vi "Test Customer Pick Up Order Broadcasts Order Item.vi"(8 "error in (no error)":errorcluster, 11 "Customer Test in":refnum<class "Customer Test.lvclass">) -> (0 "error out":errorcluster, 3 "Customer Test out":refnum<class "Customer Test.lvclass">)   [LabVIEW 2020, in "Customer Test.lvclass"]
uses:
  Customer Test.lvclass
  C:/Program Files (x86)/National Instruments/LabVIEW 2020/vi.lib/Asteme/LUnit/Test Case.lvclass
  Customer/Customer.lvclass
  C:/Program Files (x86)/National Instruments/LabVIEW 2020/vi.lib/Asteme/Triarc Framework/Process/Process.lvclass
  Support/Beverages/Beverage/Beverage.lvclass
  <vilib>/Asteme/Triarc Framework/Process/Process.lvclass/Process.ctl
  <vilib>/Asteme/LUnit/Test Case.lvclass/Test Case.ctl
  <vilib>/Asteme/LUnit/LUnit Assertion Result.lvclass/LUnit Assertion Result.ctl
  <vilib>/Asteme/Triarc Framework Test Suite/Support/Execution timer.vi
  <vilib>/Asteme/Triarc Framework/Process/Private/SubVIs/Wait for finish.vi
  <vilib>/Asteme/Triarc Framework/Process/Protected/Messaging/Enqueue Message.vi
  <vilib>/Asteme/Triarc Framework/Process/Private/SubVIs/Set Lifecycle State.vi
  <vilib>/Asteme/Triarc Framework/Process/Public/Lifecycle/Get Lifecycle State.vi
  <vilib>/Asteme/LUnit/Palette/Pass.vi
  <vilib>/Asteme/LUnit/Palette/Fail.vi
  <vilib>/Asteme/LUnit/Variant to string.vi
  <vilib>/Asteme/LUnit/Set Assertion Type.vi
  <vilib>/Utility/error.llb/Clear Errors.vi
  <vilib>/Asteme/LUnit/Add test result.vi
  <vilib>/Asteme/LUnit/LUnit Write Passed.vi
  <vilib>/Asteme/LUnit/LUnit Get Test Case.vi
  <vilib>/Asteme/LUnit/Assertion Result/LUnit Get Test Name.vi
  <vilib>/Asteme/LUnit/LUnit Write Message.vi
  <vilib>/Asteme/LUnit/LUnit Write Description.vi
  <vilib>/Asteme/LUnit/LUnit Write Assertion Type.vi
  <vilib>/Asteme/LUnit/Read Test Case Name.vi
  <vilib>/Asteme/Triarc Framework Test Suite/Support/Event Helpers/Dequeue Event Message.vi
  <vilib>/Utility/error.llb/Error Cluster From Error Code.vi
  <vilib>/Utility/Data Type/Get Type Information.vi
  <vilib>/Utility/LVClass/Get LV Class Name.vi
  <vilib>/Asteme/LUnit/LUnit Assertion Result.lvclass
  <vilib>/Asteme/Triarc Framework/Process/Process.lvclass
  <vilib>/Asteme/Triarc Framework Test Suite/Support/Event Helpers/Event Helpers.lvlib
  <vilib>/Asteme/LUnit/Test Case.lvclass
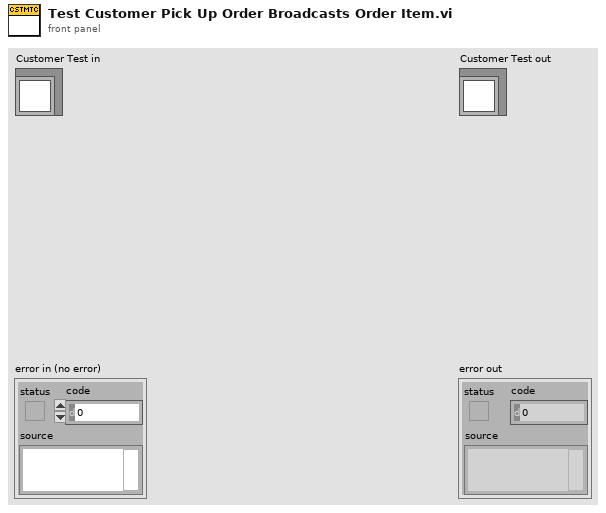
[diagram p1: front panel]
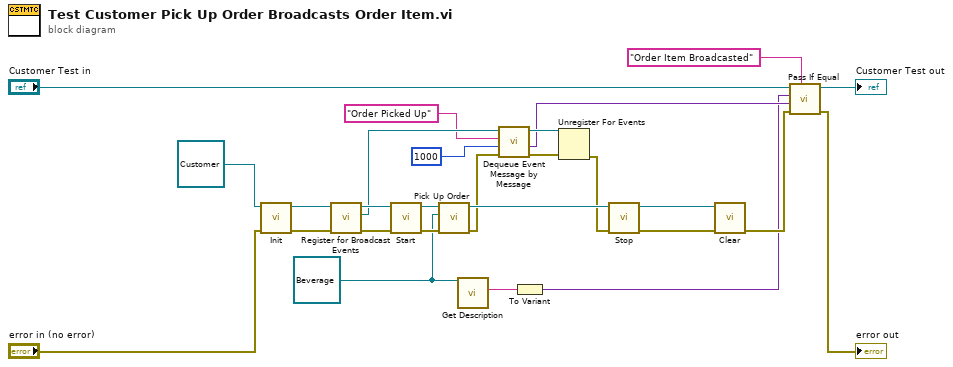
[diagram p0: block diagram]
diagram:
  w1 = refnum<class "Beverage.lvclass"> refnum ("Beverage.lvclass")
  n1 = call-dynamic "Init.vi"("error in (no error)"="error in (no error)", "View In"=refnum<class "Customer.lvclass"> refnum ("Customer.lvclass")) -> ("error out"=w23:errorcluster, "View Out"=w24:refnum<class "Customer.lvclass">)  [unwired: 8 in]
  n2 = call <vilib>:"Register for Broadcast Events.vi"("error in (no error)"=w23, "Process In"=w24) -> ("error out"=w26:errorcluster, "Event Registration Refnum Out"=w19:refnum<event-registration>, "Process Out"=w25:refnum<class "Customer.lvclass">)  [unwired: 7 in]
  n3 = call <vilib>:"Start.vi"("error in (no error)"=w26, "Process In"=w25) -> ("error out"=w16:errorcluster, "Process Out"=w18:refnum<class "Customer.lvclass">)  [unwired: 8 in]
  n4 = call-dynamic "Pick Up Order.vi"("error in (no error)"=w16, "Beverage"=w1, "Customer In"=w18) -> ("error out"=w15:errorcluster, "Customer Out"=w17:refnum<class "Customer.lvclass">)  [unwired: 7 in]
  n5 = call "Get Description.vi"("Beverage in"=w1) -> ("Description"=w2:string)  [unwired: 8 in, 2 out]
  n6 = call <vilib>:"Dequeue Event Message by Message.vi"("error in (no error)"=w15, "Timeout (-1)"=1000, "Message"="Order Picked Up", "Event Registration Refnum"=w19) -> ("error out"=w14:errorcluster, "Message Data"=w4:variant, "Event Registration Refnum Out"=w7:refnum<event-registration>)  [unwired: 3 in, 2 out]
  n7 = To Variant(anything=w2) -> (Variant=w3:variant)
  n8 = Unregister For Events(event registration refnum=w7, error in=w14) -> (error out=w11:errorcluster)
  n9 = call <vilib>:"Stop.vi"("error in (no error)"=w11, "Process In"=w17) -> ("error out"=w21:errorcluster, "Process Out"=w22:refnum<class "Customer.lvclass">)  [unwired: 7 in, 1 out]
  n10 = call-dynamic "Clear.vi"("error in (no error)"=w21, "View In"=w22) -> ("error out"=w10:errorcluster)  [unwired: 9 in]
  n11 = call <vilib>:"Pass If Equal.vi"("Description"="Order Item Broadcasted", "error in (no error)"=w10, "Actual"=w4, "Expected"=w3, "Test Case In"="Customer Test in") -> ("error out"=→"error out":errorcluster, "Test Case Out"=→"Customer Test out":refnum<class "Customer Test.lvclass">)  [unwired: 5 in]
